vi "XML - Get Channel Info from XML.vi"(8 "error in":errorcluster, 10 "XPath expression":string, 11 "Document Element Node in":refnum<k20>) -> (0 "error out":errorcluster, 2 "Channel Info":T1[](array[typedef]) {"Data Type" items=["U8", "U16", "U32", "U64", "I8", "I16", "I32", "I64", "SGL", "DBL", "EXT"]}, 3 "Document Element Node out":refnum<k20>)   [LabVIEW 2016, in "UDP-Custom-Device System Explorer.lvlib"]
uses:
  UDP-Custom-Device System Explorer.lvlib
  Types/XML/XML - Channel.ctl
  <vilib>/xml/Close Reference(Node).vi
  <vilib>/xml/Close Reference(NNMap).vi
  <vilib>/xml/NI_XML.lvlib
  <resource>/objmgr/DOMUserDefRef.rc
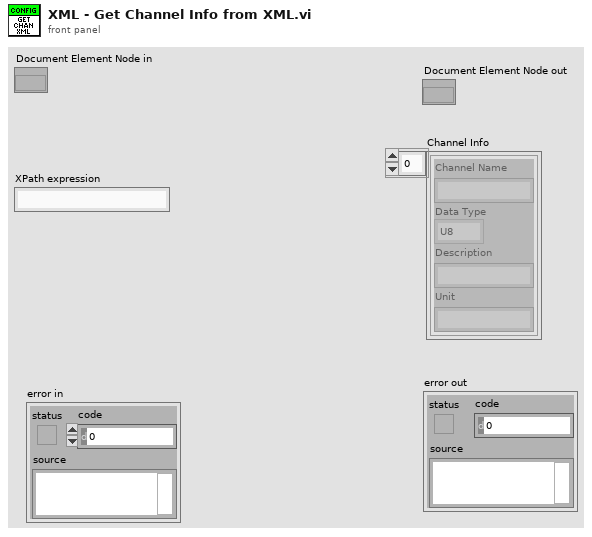
[diagram p1: front panel]
types:
  T1 = typedef "UDP-Custom-Device System Explorer.lvlib/XML - Channel.ctl" = cluster{"Channel Name":string, "Data Type":u16, "Description":string, "Unit":string}
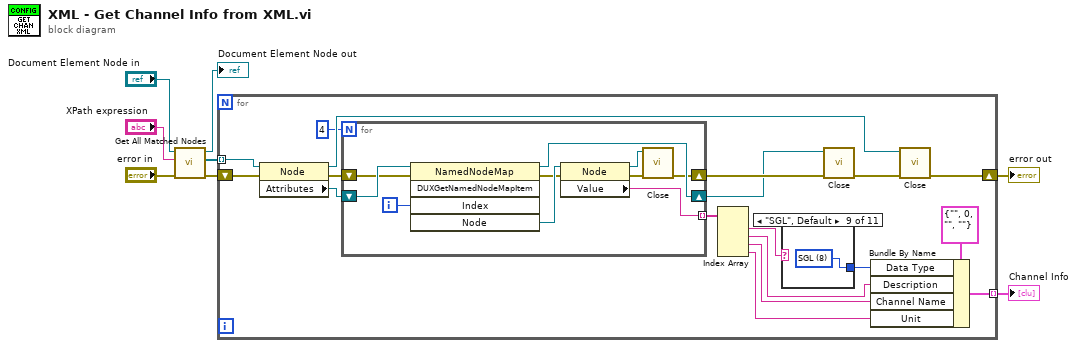
[diagram p0: block diagram]
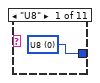
[diagram p2: hidden frame]
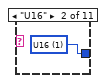
[diagram p3: hidden frame]
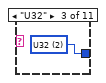
[diagram p4: hidden frame]
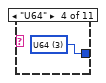
[diagram p5: hidden frame]
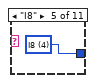
[diagram p6: hidden frame]
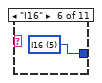
[diagram p7: hidden frame]
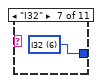
[diagram p8: hidden frame]
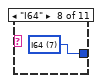
[diagram p9: hidden frame]
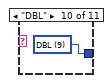
[diagram p10: hidden frame]
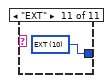
[diagram p11: hidden frame]
diagram:
  n1 = call <vilib>:"Get All Matched Nodes.vi"("error in (no error)"="error in", "XPath expression"="XPath expression", "node in"="Document Element Node in") -> ("error out"=w7:errorcluster, "node result array"=w6:refnum<k20>[], "node out"=→"Document Element Node out":refnum<k20>)  [unwired: 6 in]
  n2 = for {
    tunnel: w6 -> [w25] mode=indexing
    shift-right: [w20] -> w8
    shift-left: w7 -> [w26]
    tunnel: [w12] -> w1 mode=indexing
    n3 = property class="Node"(reference=w25, error in=w26) -> (reference out=w21:refnum<k20>, error out=w23:errorcluster, "Attributes"=w24:refnum<k20>)
    n4 = for {
      N: 4 -> [_]
      tunnel: [w42] -> w19 mode=indexing
      shift-right: [w38] -> w17
      shift-left: w23 -> [w46]
      shift-right: [w43] -> w11
      shift-left: w24 -> [w47]
      i -> [w41]
      n5 = invoke class="NamedNodeMap" method="DUXGetNamedNodeMapItem"(reference=w47, error in=w46, "Index"=w41) -> (reference out=w43:refnum<k20>, error out=w44:errorcluster, "Node"=w45:refnum<k20>)  [unwired: 2 in, 2 out]
      n6 = property class="Node"(reference=w45, error in=w44) -> (reference out=w40:refnum<k20>, error out=w39:errorcluster, "Value"=w42:string)
      n7 = call-poly <vilib>:"Close.vi"("error in (no error)"=w39, "node"=w40) -> ("error out"=w38:errorcluster)  [unwired: 7 in]
    }
    n8 = Index Array(array=w19) -> (element #1=w10:string, element #2=w15:string, element #3=w14:string, element #4=w13:string)  [unwired: 4 in]
    n9 = case shown="\"SGL\", Default" w10 {
      tunnel: [w27 w28 w29 w30 w31 w32 w33 w34 w35 w36 w37] -> w9
      frame "U8" {
        w27 = u16 0 items=["U8", "U16", "U32", "U64", "I8", "I16", "I32", "I64", "SGL", "DBL", "EXT"] ("Data Type")
      }
      frame "U16" {
        w28 = u16 1 items=["U8", "U16", "U32", "U64", "I8", "I16", "I32", "I64", "SGL", "DBL", "EXT"] ("Data Type")
      }
      frame "U32" {
        w29 = u16 2 items=["U8", "U16", "U32", "U64", "I8", "I16", "I32", "I64", "SGL", "DBL", "EXT"] ("Data Type")
      }
      frame "U64" {
        w30 = u16 3 items=["U8", "U16", "U32", "U64", "I8", "I16", "I32", "I64", "SGL", "DBL", "EXT"] ("Data Type")
      }
      frame "I8" {
        w31 = u16 4 items=["U8", "U16", "U32", "U64", "I8", "I16", "I32", "I64", "SGL", "DBL", "EXT"] ("Data Type")
      }
      frame "I16" {
        w32 = u16 5 items=["U8", "U16", "U32", "U64", "I8", "I16", "I32", "I64", "SGL", "DBL", "EXT"] ("Data Type")
      }
      frame "I32" {
        w33 = u16 6 items=["U8", "U16", "U32", "U64", "I8", "I16", "I32", "I64", "SGL", "DBL", "EXT"] ("Data Type")
      }
      frame "I64" {
        w34 = u16 7 items=["U8", "U16", "U32", "U64", "I8", "I16", "I32", "I64", "SGL", "DBL", "EXT"] ("Data Type")
      }
      frame "SGL", Default {
        w35 = u16 8 items=["U8", "U16", "U32", "U64", "I8", "I16", "I32", "I64", "SGL", "DBL", "EXT"] ("Data Type")
      }
      frame "DBL" {
        w36 = u16 9 items=["U8", "U16", "U32", "U64", "I8", "I16", "I32", "I64", "SGL", "DBL", "EXT"] ("Data Type")
      }
      frame "EXT" {
        w37 = u16 10 items=["U8", "U16", "U32", "U64", "I8", "I16", "I32", "I64", "SGL", "DBL", "EXT"] ("Data Type")
      }
    }
    n10 = call-poly <vilib>:"Close.vi"("error in (no error)"=w17, "named node map"=w11) -> ("error out"=w22:errorcluster)  [unwired: 7 in]
    n11 = Bundle By Name(cluster=T1 {"Channel Name"="", "Data Type"=0, "Description"="", "Unit"=""} ("Channel"), "Data Type"=w9, "Description"=w15, "Channel Name"=w14, "Unit"=w13) -> (w12:T1)
    n12 = call-poly <vilib>:"Close.vi"("error in (no error)"=w22, "node"=w21) -> ("error out"=w20:errorcluster)  [unwired: 7 in]
  }
  "error out" <- w8
  "Channel Info" <- w1
